vi "Query Calibration kits.vi"(8 "error in (no error)":errorcluster, 10 "Connector type":T1(ring), 11 "VNA-Keysight PNA in":refnum<class "VNA-Keysight PNA.lvclass">) -> (0 "error out":errorcluster, 2 "Cal kits installed":string[](array[string]), 3 "VNA-Keysight PNA out":refnum<class "VNA-Keysight PNA.lvclass">)   [LabVIEW 2020, in "VNA-Keysight PNA.lvclass"]
doc: "Queryes the calibration kits installed on the VNA dependent on connector type.\nIf the VNA support E-cal it reports this aswell as the first sting in the array."
uses:
  VNA-Keysight PNA.lvclass
  C:/Sandbox/Git_Sandbox/WiSpry Test Framework source code (LV20)/WiSpry Test Framework/Instruments/Instrument.lvclass
  Instrument.lvclass/Instrument.ctl
  Instrument.lvclass
  <instrlib>/Keysight PNA Series/Keysight PNA Series.lvlib
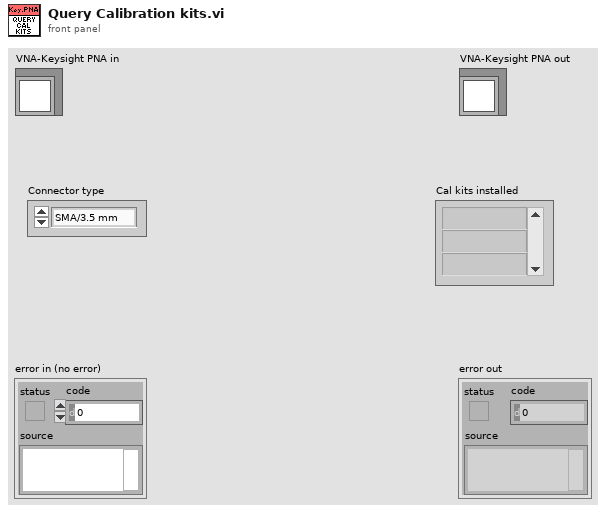
[diagram p1: front panel]
types:
  T1 = enum16{"SMA/3.5 mm", "2.92 mm", "2.4 mm", "1.85 mm", "N 50 Ohm", "N 75 Ohm", "7-16"}
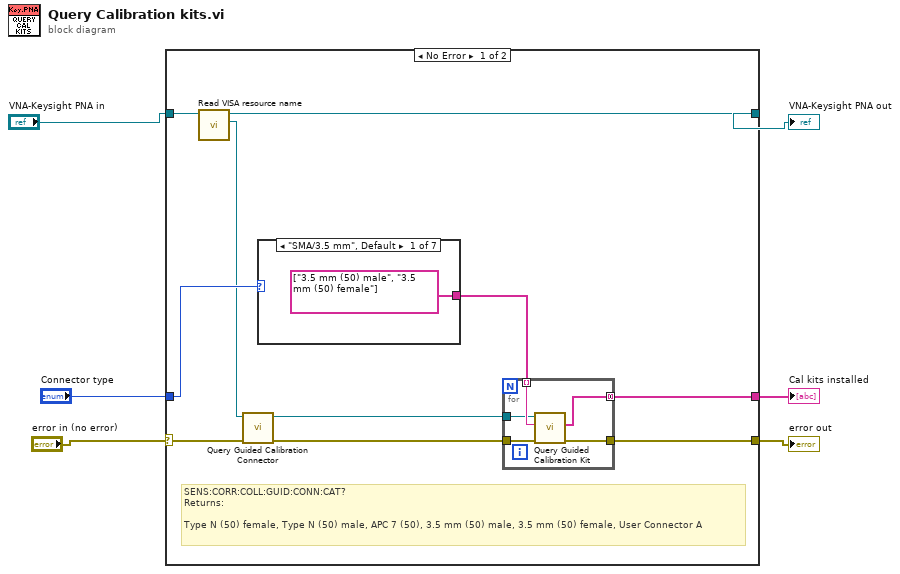
[diagram p0: block diagram]
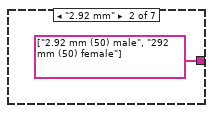
[diagram p2: hidden frame]
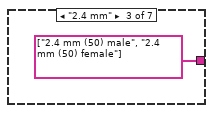
[diagram p3: hidden frame]
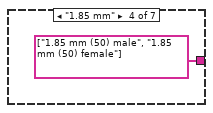
[diagram p4: hidden frame]
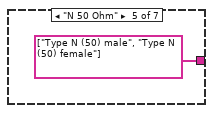
[diagram p5: hidden frame]
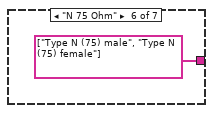
[diagram p6: hidden frame]
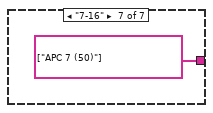
[diagram p7: hidden frame]
diagram:
  n1 = case shown="No Error" "error in (no error)" {
    selector: "error in (no error)" -> [w14 w29]
    tunnel: [w15 w30] -> w4
    tunnel: "VNA-Keysight PNA in" -> [w16 w30]
    tunnel: [w12 w29] -> w3
    tunnel: "Connector type" -> [w13 _]
    tunnel: [w8 _] -> w1
    frame No Error {
      # "SENS:CORR:COLL:GUID:CONN:CAT?\nReturns:\n\nType N (50) female, Type N (50) male, APC 7 (50), 3.5 mm (50) male, 3.5 mm (50) female, User Connector A"
      n2 = call "Read VISA resource name.vi"("Instrument in"=w16) -> ("VISA resource name"=w7:refnum<visa-resource-name>, "Instrument out"=w15:refnum<class "VNA-Keysight PNA.lvclass">)  [unwired: 9 in]
      n3 = call <instrlib>:"Query Guided Calibration Connector.vi"("error in (no error)"=w14, "VISA resource name"=w7) -> ("error out"=w9:errorcluster, "VISA resource name out"=w10:refnum<visa-resource-name>)  [unwired: 7 in, 1 out]
      n4 = case shown="\"SMA/3.5 mm\", Default" w13 {
        tunnel: [string[] ["3.5 mm (50) male", "3.5 mm (50) female"] string[] ["2.92 mm (50) male", "292 mm (50) female"] string[] ["2.4 mm (50) male", "2.4 mm (50) female"] string[] ["1.85 mm (50) male", "1.85 mm (50) female"] string[] ["Type N (50) male", "Type N (50) female"] string[] ["Type N (75) male", "Type N (75) female"] string[] ["APC 7 (50)"]] -> w11
        frame "SMA/3.5 mm", Default {
        }
        frame "2.92 mm" {
        }
        frame "2.4 mm" {
        }
        frame "1.85 mm" {
        }
        frame "N 50 Ohm" {
        }
        frame "N 75 Ohm" {
        }
        frame "7-16" {
        }
      }
      n5 = for {
        tunnel: [w21] -> w12
        tunnel: w11 -> [w20] mode=indexing
        tunnel: w10 -> [w19]
        tunnel: w9 -> [w18]
        tunnel: [w17] -> w8 mode=concatenating
        n6 = call <instrlib>:"Query Guided Calibration Kit.vi"("error in (no error)"=w18, "Connector ('Not used')"=w20, "VISA resource name"=w19) -> ("error out"=w21:errorcluster, "Calibration Kits"=w17:string[])  [unwired: 6 in, 1 out]
      }
    }
    frame Error {
    }
  }
  "error out" <- w3
  "VNA-Keysight PNA out" <- w4
  "Cal kits installed" <- w1
